vi "Shutdown.vi"(8 "error in (no error)":errorcluster, 11 "LogEngine.lvclass":refnum<class "LogEngine.lvclass">) -> (0 "error out":errorcluster, 3 "LogEngine.lvclass":refnum<class "LogEngine.lvclass">)   [LabVIEW 2017, in "LogEngine.lvclass"]
doc: "Developed by Kevin Thompson\nkevin@thompsonengineering.net\n\nCopyright 2018-2020\nThompson Engineering, LLC"
uses:
  LogEngine.lvclass
  LogEngine.lvclass/LogEngine.ctl
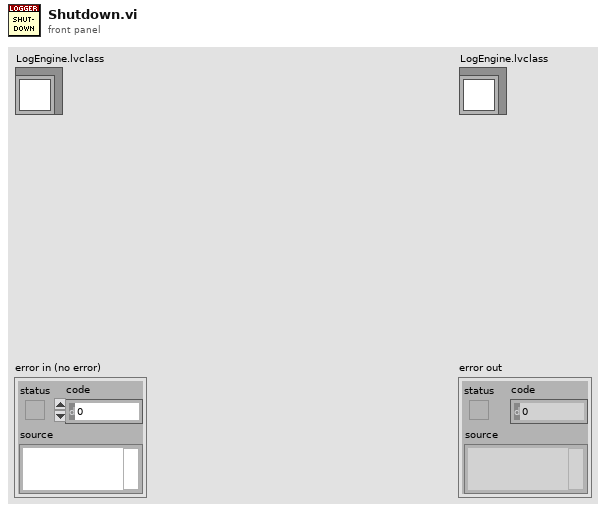
[diagram p1: front panel]
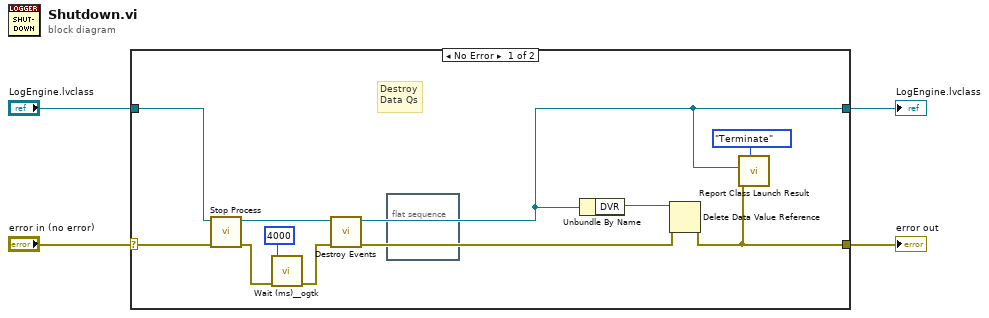
[diagram p0: block diagram]
diagram:
  n1 = case shown="No Error" "error in (no error)" {
    selector: "error in (no error)" -> [w9 w17]
    tunnel: [w8 w17] -> w3
    tunnel: [w11 w16] -> w1
    tunnel: "LogEngine.lvclass" -> [w15 w16]
    frame No Error {
      # "Destroy\nData Qs"
      n2 = call "Stop Process.vi"("error in (no error)"=w9, "LogEngine.lvclass"=w15) -> ("error out"=w7:errorcluster, "LogEngine.lvclass"=w14:refnum<class "LogEngine.lvclass">)  [unwired: 8 in]
      n3 = call <userlib>:"Wait (ms)__ogtk.vi"("error in (no error)"=w7, "milliseconds to wait"=u32 4000) -> ("error out"=w6:errorcluster)  [unwired: 8 in, 1 out]
      n4 = call "Destroy Events.vi"("error in (no error)"=w6, "LogEngine.lvclass"=w14) -> ("error out"=w10:errorcluster, "LogEngine.lvclass"=w11:refnum<class "LogEngine.lvclass">)  [unwired: 8 in]
      n5 = flat-sequence {
        frame #0 {
        }
      }
      n6 = Unbundle By Name(w11) -> ("DVR"=w13:refnum<data-value>)
      n7 = Delete Data Value Reference(data value reference=w13, error in=w10) -> (error out=w8:errorcluster)  [unwired: 1 out]
      n8 = call "Report Class Launch Result.vi"("Object"=w11, "error in (no error)"=w8, "Mode (Launch)"=enum16{"Launch", "Terminate"}."Terminate") -> ()  [unwired: 7 in, 1 out]
    }
    frame Error {
    }
  }
  "error out" <- w3
  "LogEngine.lvclass" <- w1
